vi "总磷总氮量程写入.vi"(7 "error in (no error)":errorcluster caption="错误输入（无错误）", 9 "量程参数写入":T1, 10 "测量参数":u16(ring) items=["COD"=22, "氨氮"=3, "总氮"=2, "总磷"=1]) -> (0 "error out":errorcluster caption="错误输出")   [LabVIEW 2016, in "斯坦道氟化物.lvlib"]
panel:
  out "输出数组":u16[](array[numeric]) format="%04x"
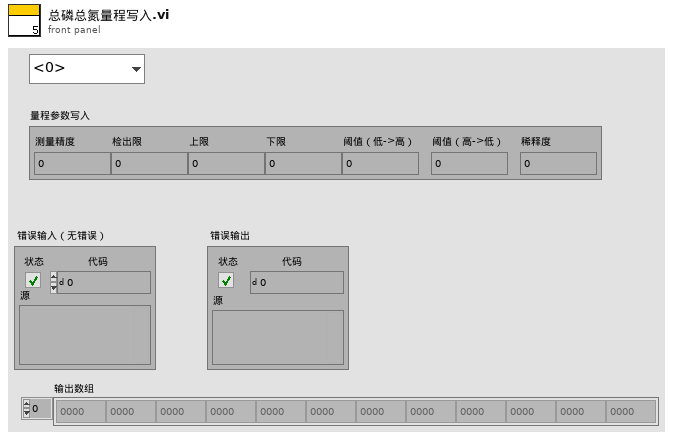
[diagram p1: front panel]
types:
  T1 = cluster{"测量精度":u16, "检出限":dbl, "上限":dbl, "下限":dbl, "阈值（低->高）":dbl, "阈值（高->低）":dbl, "稀释度":dbl}
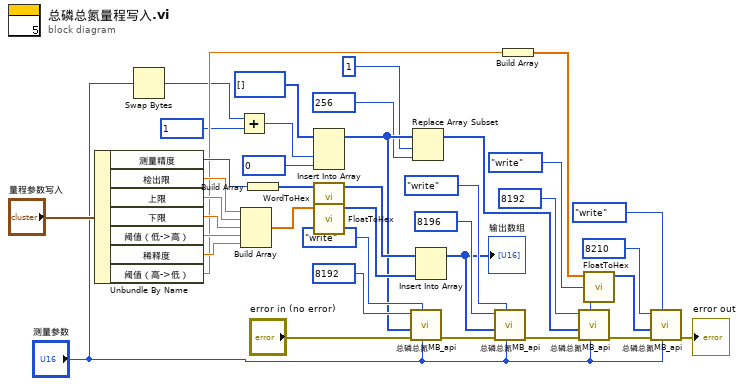
[diagram p0: block diagram]
diagram:
  n1 = Unbundle By Name("量程参数写入") -> ("测量精度"=w21:u16, "检出限"=w20:dbl, "上限"=w19:dbl, "下限"=w18:dbl, "阈值（低->高）"=w17:dbl, "稀释度"=w16:dbl, "阈值（高->低）"=w11:dbl)
  n2 = Swap Bytes(anything="测量参数") -> (byte swapped=w2:u16)
  n3 = Add(x=w2, y=u16 1 ("starting address")) -> (x+y=w8:u16)
  n4 = Build Array(w20, w19, w18, w17, w16) -> (w15:dbl[])
  n5 = Build Array(w21) -> (w22:u16[])
  n6 = Insert Into Array(array=u16[] [] ("数组"), new element #1=w8, new element #2=u16 0 ("starting address")) -> (w7:u16[])  [unwired: 1 in]
  n7 = call "WordToHex.vi"("WORD"=w22) -> ("数组"=w14:u16[])  [unwired: 10 in]
  n8 = call "FloatToHex.vi"("浮点数"=w15) -> ("DCBA整形输出"=w13:u16[])  [unwired: 10 in]
  n9 = call "总磷总氮MB_api.vi"("Slave ID"="测量参数", "STEP"=enum16{"open", "read", "write", "close"}."write", "Error in"="error in (no error)", "values"=w7, "starting address"=u16 8192) -> ("error out"=w33:errorcluster)  [unwired: 4 in, 2 out]
  n10 = Replace Array Subset(array=w7, new element=u16 256 ("starting address"), index=1 ("索引")) -> (w5:u16[])
  n11 = Insert Into Array(array=w14, new element=w13) -> (w12:u16[])  [unwired: 1 in]
  "输出数组" <- w12
  n12 = call "总磷总氮MB_api.vi"("Slave ID"="测量参数", "STEP"=enum16{"open", "read", "write", "close"}."write", "Error in"=w33, "values"=w12, "starting address"=u16 8196) -> ("error out"=w30:errorcluster)  [unwired: 4 in, 2 out]
  n13 = Build Array(w11) -> (w10:dbl[])
  n14 = call "总磷总氮MB_api.vi"("Slave ID"="测量参数", "STEP"=enum16{"open", "read", "write", "close"}."write", "Error in"=w30, "values"=w5, "starting address"=u16 8192) -> ("error out"=w29:errorcluster)  [unwired: 4 in, 2 out]
  n15 = call "FloatToHex.vi"("浮点数"=w10) -> ("DCBA整形输出"=w9:u16[])  [unwired: 10 in]
  n16 = call "总磷总氮MB_api.vi"("Slave ID"="测量参数", "STEP"=enum16{"open", "read", "write", "close"}."write", "Error in"=w29, "values"=w9, "starting address"=u16 8210) -> ("error out"=→"error out":errorcluster)  [unwired: 4 in, 2 out]
